vi "Interpolate (1 point 1 Channel).vi"(8 "Data Valid":bool=TRUE, 9 "x[n].ResampleInfo":T3, 10 "Current Point.Value":T4 format="%.16g", 11 "Previous Point.Value":T4 format="%.6f") -> (3 "Output Data":T2)   [LabVIEW 2011]
doc: "This VI performs a linear interporation between two points using DSP48E.\n\n<b> Lambda </b> is the distance between the previous point and required interpolation point\n\n<b> Latency = 6 Ticks <\\b>"
uses:
  <userlib>/FPGA Library/Code Development/Signal Processing/Interpolation Block/Controls/Interpolation Input Data.ctl
  <userlib>/FPGA Library/Code Development/Signal Processing/Interpolation Block/Controls/ResampleVectorInfo (Single Point).ctl
  <userlib>/FPGA Library/Code Development/Signal Processing/Interpolation Block/Controls/Interpolation Output Data.ctl
  <vilib>/rvi/FXPMathLib/FxpConvert/subVIs/nifxpmath_Convert_SimConfig.ctl
  <vilib>/fxp/LVFixedPointQuantizationPolicyTypeDef.ctl
  <vilib>/fxp/LVFixedPointOverflowPolicyTypeDef.ctl
  <vilib>/rvi/FXPMathLib/FxpSub/subVIs/nifxpmath_Sub_SimConfig.ctl
  <vilib>/rvi/FXPMathLib/basic elements/DSP48E/simVIs/niFpgaDsp48eRegisters.ctl
  <vilib>/rvi/FXPMathLib/basic elements/DSP48E/simVIs/niFpgaDsp48eEnables.ctl
  <vilib>/rvi/FXPMathLib/basic elements/DSP48E/simVIs/niFpgaDsp48eResets.ctl
  <vilib>/rvi/FXPMathLib/basic elements/DSP48E/simVIs/niFpgaDsp48eSimulationState.ctl
  <vilib>/rvi/FXPMathLib/basic elements/DSP48E/subVIs/niFpgaDsp48eType.ctl
  <vilib>/rvi/FXPMathLib/basic elements/DSP48E/subVIs/niFpgaDsp48eAlumodeOpmodeCarryinselState.ctl
  <vilib>/rvi/FXPMathLib/basic elements/DSP48E/subVIs/niFpgaDsp48eUseMultiplierState.ctl
  <vilib>/rvi/FXPMathLib/basic elements/DSP48E/subVIs/niFpgaDsp48eLogicUnitModeState.ctl
  <vilib>/rvi/FXPMathLib/basic elements/DSP48E/subVIs/niFpgaDsp48eSelectPatternState.ctl
  <vilib>/rvi/FXPMathLib/basic elements/DSP48E/subVIs/niFpgaDsp48eSelectMaskState.ctl
  <vilib>/rvi/FXPMathLib/basic elements/DSP48E/subVIs/niFpgaDsp48eAutoresetState.ctl
  <vilib>/rvi/FXPMathLib/FxpConvert/simVIs/DllFxpConvertTemp_sub.vi
  <vilib>/rvi/FXPMathLib/FxpSub/simVIs/DllFxpSubTemp_sub.vi
  <vilib>/rvi/FXPMathLib/basic elements/DSP48E/simVIs/niFpgaDsp48eSimMultiplier.vi
  <vilib>/rvi/FXPMathLib/basic elements/DSP48E/simVIs/niFpgaDsp48eSimArithmetic.vi
  <vilib>/rvi/FXPMathLib/basic elements/DSP48E/simVIs/niFpgaDsp48eSimPatternDetect.vi
  <vilib>/rvi/FXPMathLib/basic elements/DSP48E/simVIs/niFpgaDsp48eSimP.vi
  <vilib>/rvi/FXPMathLib/basic elements/DSP48E/simVIs/niFpgaDsp48eSimUpdateState.vi
  <vilib>/rvi/FXPMathLib/basic elements/DSP48E/simVIs/niFpgaDsp48eCheckMode.vi
  <vilib>/rvi/FXPMathLib/basic elements/DSP48E/simVIs/niFpgaDsp48eReportInvalidMode.vi
  <vilib>/rvi/FXPMathLib/basic elements/FxpDiscreteDelay/XNode/nifxpmath_DiscreteDelay.xnode
  <vilib>/rvi/FXPMathLib/FxpConvert/XNode/nifxpmath_Convert.xnode
  <vilib>/rvi/FXPMathLib/FxpInterpret/XNode/nifxpmath_Interpret.xnode
  <vilib>/rvi/FXPMathLib/FxpSub/XNode/nifxpmath_Sub.xnode
  <vilib>/rvi/FXPMathLib/basic elements/DSP48E/XNode/niFpgaDsp48e.xnode
panel:
  out "Interpolation Overflow":bool
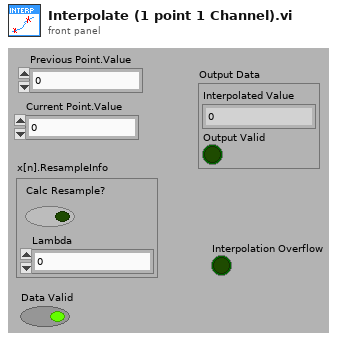
[diagram p1: front panel]
types:
  T1 = typedef "Interpolation Output Data.ctl" = fxp<+/-,19,1>
  T2 = cluster{"Interpolated Value":T1, "Output Valid":bool}
  T3 = typedef "ResampleVectorInfo (Single Point).ctl" = cluster{"Calc Resample?":bool, "Lambda":fxp<+/-,18,1>}
  T4 = typedef "Interpolation Input Data.ctl" = fxp<+/-,18,1>
  T5 = cluster{"Calc Resample?":bool, "Lambda":fxp<+/-,18,1>}
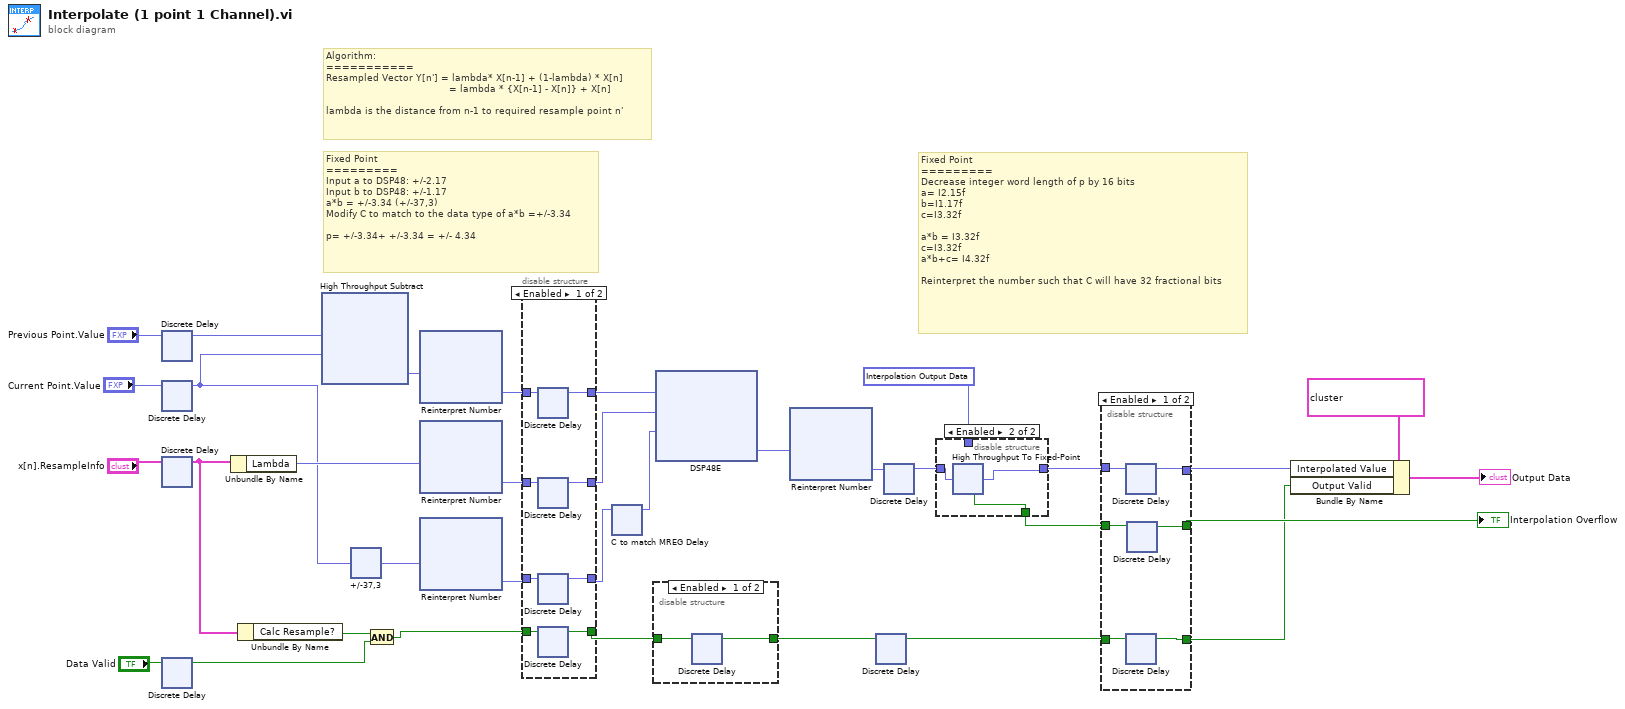
[diagram p0: block diagram]
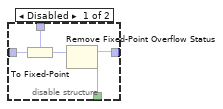
[diagram p2: hidden frame]
diagram:
  # "Algorithm:\n===========\nResampled Vector Y[n'] = lambda* X[n-1] + (1-lambda) * X[n]\n                                         = lambda * {X[n-1] - X[n]} + X[n]\n\nlambda is the distance from n-1 to required resample point n'"
  # "Fixed Point\n=========\nDecrease integer word length of p by 16 bits\na= I2.15f\nb=I1.17f\nc=I3.32f\n\na*b = I3.32f\nc=I3.32f\na*b+c= I4.32f\n\nReinterpret the number such that C will have 32 fractional bits"
  # "Fixed Point\n=========\nInput a to DSP48: +/-2.17\nInput b to DSP48: +/-1.17 \na*b = +/-3.34 (+/-37,3)\nModify C to match to the data type of a*b =+/-3.34\n\np= +/-3.34+ +/-3.34 = +/- 4.34"
  n1 = xnode "Discrete Delay"("D"="Previous Point.Value") -> ("Q"=w10:fxp<+/-,18,1>)
  n2 = xnode "Discrete Delay"("D"="Current Point.Value") -> ("Q"=w9:fxp<+/-,18,1>)
  n3 = xnode "Discrete Delay"("D"="x[n].ResampleInfo") -> ("Q"=w8:T5)
  n4 = xnode "Discrete Delay"("D"="Data Valid") -> ("Q"=w7:bool)
  n5 = Unbundle By Name(w8) -> ("Lambda"=w19:fxp<+/-,18,1>)
  n6 = Unbundle By Name(w8) -> ("Calc Resample?"=w13:bool)
  n7 = xnode "High Throughput Subtract"("x"=w10, "y"=w9) -> ("x-y"=w34:fxp<+/-,19,2>)
  n8 = xnode "+/-37,3"("x"=w9) -> ("y"=w27:fxp<+/-,37,3>)
  n9 = And(x=w13, y=w7) -> (x .and. y?=w11:bool)
  n10 = xnode "Reinterpret Number"("x"=w34) -> ("y"=w33:fxp<+/-,19,19>)
  n11 = xnode "Reinterpret Number"("x"=w19) -> ("y"=w32:fxp<+/-,18,18>)
  n12 = xnode "Reinterpret Number"("x"=w27) -> ("y"=w29:fxp<+/-,37,37>)
  n13 = disable-structure shown="Enabled" {
    disable-tunnel: w33 -> [w42 w46]
    disable-tunnel: w32 -> [w41 w45]
    disable-tunnel: w29 -> [w40 w44]
    disable-tunnel: w11 -> [w39 w43]
    disable-tunnel: [w38 w43] -> w21
    disable-tunnel: [w37 w44] -> w6
    disable-tunnel: [w36 w45] -> w23
    disable-tunnel: [w35 w46] -> w22
    frame Enabled {
      n14 = xnode "Discrete Delay"("D"=w42) -> ("Q"=w35:fxp<+/-,19,19>)
      n15 = xnode "Discrete Delay"("D"=w41) -> ("Q"=w36:fxp<+/-,18,18>)
      n16 = xnode "Discrete Delay"("D"=w40) -> ("Q"=w37:fxp<+/-,37,37>)
      n17 = xnode "Discrete Delay"("D"=w39) -> ("Q"=w38:bool)
    }
    frame Disabled {
      # "Disable\nZ nodes\nfor sim"
    }
  }
  n18 = xnode "C to match MREG Delay"("D"=w6) -> ("Q"=w5:fxp<+/-,37,37>)
  n19 = disable-structure shown="Enabled" {
    disable-tunnel: w21 -> [w48 w49]
    disable-tunnel: [w47 w49] -> w20
    frame Enabled {
      n20 = xnode "Discrete Delay"("D"=w48) -> ("Q"=w47:bool)
    }
    frame Disabled {
      # "Disable\nZ nodes for sim"
    }
  }
  n21 = xnode "DSP48E"("a"=w22, "b"=w23, "c"=w5) -> ("p"=w31:fxp<+/-,48,48>)
  n22 = xnode "Reinterpret Number"("x"=w31) -> ("y"=w28:fxp<+/-,48,14>)
  n23 = xnode "Discrete Delay"("D"=w20) -> ("Q"=w4:bool)
  n24 = xnode "Discrete Delay"("D"=w28) -> ("Q"=w3:fxp<+/-,48,14>)
  n25 = disable-structure shown="Enabled" {
    disable-tunnel: [w51 w56] -> w2
    disable-tunnel: T1 0.0 ("Interpolate.Input Data") -> [w54 _]
    disable-tunnel: w3 -> [w53 w57]
    disable-tunnel: [w50 w55] -> w1
    frame Disabled {
      n26 = To Fixed-Point(fixed-point type=w54, number=w53) -> (fixed-point=w52:T1)
      n27 = Remove Fixed-Point Overflow Status(3:w52) -> (0:w50:bool, 1:w51:T1)
    }
    frame Enabled {
      n28 = xnode "High Throughput To Fixed-Point"("x"=w57) -> ("y"=w56:fxp<+/-,19,1>, "operation overflow"=w55:bool)
    }
  }
  n29 = disable-structure shown="Enabled" {
    disable-tunnel: w1 -> [w81 w88]
    disable-tunnel: w2 -> [w86 w89]
    disable-tunnel: w4 -> [w83 w87]
    disable-tunnel: [w85 w89] -> w15
    disable-tunnel: [w84 w88] -> w24
    disable-tunnel: [w82 w87] -> w14
    frame Enabled {
      n30 = xnode "Discrete Delay"("D"=w86) -> ("Q"=w85:fxp<+/-,19,1>)
      n31 = xnode "Discrete Delay"("D"=w83) -> ("Q"=w82:bool)
      n32 = xnode "Discrete Delay"("D"=w81) -> ("Q"=w84:bool)
    }
    frame Disabled {
      # "Disable\nZ nodes\nfor sim"
    }
  }
  "Interpolation Overflow" <- w24
  n33 = Bundle By Name(cluster=T2 {"Interpolated Value"=0.0, "Output Valid"=FALSE} ("Cluster"), "Interpolated Value"=w15, "Output Valid"=w14) -> (→"Output Data":T2)
